vi "Get Integer Coefficients of Fixed-Point FIR Filter.vi"() -> ()   [LabVIEW 2023]
doc: "Demonstrates how to use the DFD Convert FXP to Integer VI to get integer coefficients of a fixed-point finite impulse response (FIR) filter.\n\nCompete the following steps to use this VI.\n1) Configure the <B>Coefficient Quantizer</B>.\n2) Run the VI.\n3) Observe the Coefficients Report.\n4) Examine the block diagram to learn how to get integer coefficients of a fixed-point FIR filter."
uses:
  <vilib>/addons/Digital Filter Design/_Objects.llb/DFD Quantization Settings.ctl
  <vilib>/addons/Digital Filter Design/_Objects.llb/DFD Quantization Sources.ctl
  <vilib>/addons/Digital Filter Design/FXPModel.llb/DFD FXP Quantize Coef (Advanced).vi
  <vilib>/addons/Digital Filter Design/FXPModel.llb/DFD FXP Get Quantizer (One).vi
  <vilib>/addons/Digital Filter Design/FXPLib.llb/DFD FXP to I16 (vector).vi
  <vilib>/addons/Digital Filter Design/NI_DigFilterLicensed.lvlib
panel:
  out "Coefficients Report":string
  out "Floating-Point FIR Coefficients":dbl[](array[numeric])
  out "Fixed-Point FIR Coefficients":dbl[](array[numeric])
  out "I16 FIR Coefficients":i16[](array[numeric])
  in  "Coefficients Quantizer":T1={"source"=7, "wl"=16, "iwl"=1, "overflow mode"=enum."Saturation", "rounding mode"=enum."Nearest", "signed?"=TRUE} {"source" items=["Coefficients a/k"=0, "Coefficients b/v"=7, "Input"=1, "Output"=2, "Multiplicand"=3, "Product"=4, "Sum"=5, "Delay"=6]}
  # "Select Help>>Show Context Help and move the cursor over the VI icon for more information."
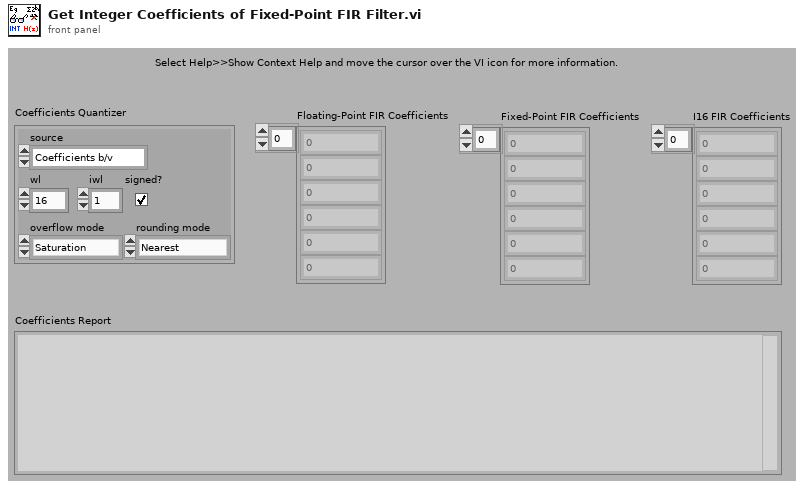
[diagram p1: front panel]
types:
  T1 = typedef "NI_DigFilterLicensed.lvlib/DFD Quantization Settings.ctl" = cluster{"source":T2, "wl":i16, "iwl":i16, "overflow mode":enum16{"Saturation", "Wrap"}, "rounding mode":enum16{"Nearest", "Truncation"}, "signed?":bool}
  T2 = typedef "NI_DigFilterLicensed.lvlib/DFD Quantization Sources.ctl" = u16
  T3 = typedef "NI_DigFilterLicensed.lvlib/DFD Filter Obj.ctl" = cluster{"mSRate_Fs":dbl, "mSRate_Version":string, "mSRate_Comments":string, "mSRate_OrgCoef":T4, "mSRate_CurCoef":T4, "mSRate_Quantized?":bool, "mSRate_QCoef":T4, "mSRate_QSettings":T6[], "mSRate_Order":i32, "mSRate_Scaling":cluster{"mSRate_ScaleByPowerOf2?":bool, "mSRate_ScaleType":T8}}
  T4 = typedef "NI_DigFilterLicensed.lvlib/DFD Filter Coef.ctl" = cluster{"type":T5, "gain":dbl, "coef a (k)":dbl[], "coef b (v)":dbl[]}
  T5 = typedef "NI_DigFilterLicensed.lvlib/DFD Filter Structure Type Selector.ctl" = enum16{"Undefined", "FIR Direct Form", "FIR Direct Form Transposed", "FIR Symmetric", "FIR Antisymmetric", "IIR Direct Form I", "IIR Direct Form I Transposed", "IIR Direct Form II", "IIR Direct Form II Transposed", "IIR Cascaded Second Order Sections Form I", "IIR Cascaded Second Order Sections Form I Transposed", "IIR Cascaded Second Order Sections Form II", "IIR Cascaded Second Order Sections Form II Transposed", "Lattice Allpass (basic sections)", "Lattice Allpass (one multiplier sections)", "Lattice Allpass (normalized sections)", "Lattice AR (basic sections)", "Lattice AR (one multiplier sections)", "Lattice AR (normalized sections)", "Lattice MA (minimum phase)", "Lattice MA (maximum phase)", "Lattice ARMA (basic sections)", "Lattice ARMA (one multiplier sections)", "Lattice ARMA (normalized sections)"}
  T6 = typedef "NI_DigFilterLicensed.lvlib/dfd_Internal Quantization Settings.ctl" = cluster{"source":T7, "wl":i16, "iwl":i16, "overflow mode":enum16{"Saturation", "Wrap"}, "rounding mode":enum16{"Nearest", "Truncation"}, "signed?":bool}
  T7 = typedef "NI_DigFilterLicensed.lvlib/dfd_Internal Quantization Srcs.ctl" = u16
  T8 = typedef "NI_DigFilterLicensed.lvlib/DFD Coef Norm Type.ctl" = enum16{"No Norm", "Time Domain 1-Norm", "Time Domain 2-Norm", "Time Domain Inf-Norm"}
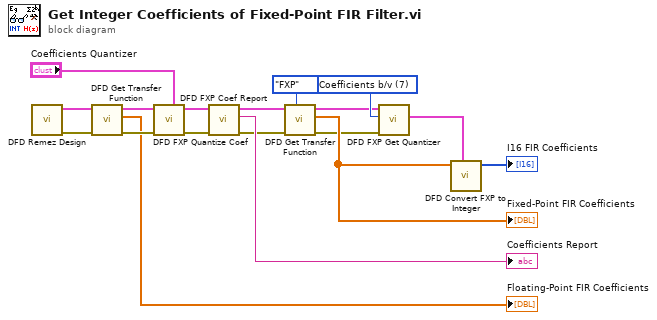
[diagram p0: block diagram]
diagram:
  w4 = T2 7 items=["Coefficients a/k"=0, "Coefficients b/v"=7, "Input"=1, "Output"=2, "Multiplicand"=3, "Product"=4, "Sum"=5, "Delay"=6] ("quantizer source")
  n1 = call <vilib>:"DFD Remez Design.vi"() -> ("error out"=w14:errorcluster, "filter out"=w15:T3)  [unwired: 7 in, 3 out]
  n2 = call <vilib>:"DFD Get Transfer Function.vi"("error in (no error)"=w14, "filter in"=w15) -> ("error out"=w12:errorcluster, "numerator"=→"Floating-Point FIR Coefficients":dbl[], "filter out"=w13:T3)  [unwired: 7 out]
  n3 = call-poly <vilib>:"DFD FXP Quantize Coef.vi"("coefficients b/v quantizer"="Coefficients Quantizer", "error in (no error)"=w12, "filter in"=w13) -> ("error out"=w9:errorcluster, "filter out"=w10:T3)  [unwired: 2 in, 5 out]
  n4 = call <vilib>:"DFD FXP Coef Report.vi"("error in (no error)"=w9, "filter in"=w10) -> ("error out"=w6:errorcluster, "coefficients report"=→"Coefficients Report":string, "filter out"=w7:T3)  [unwired: 7 out]
  n5 = call <vilib>:"DFD Get Transfer Function.vi"("type (FLP)"=enum16{"FLP", "FXP"}."FXP", "error in (no error)"=w6, "filter in"=w7) -> ("error out"=w5:errorcluster, "numerator"=w17:dbl[], "filter out"=w3:T3)  [unwired: 6 out]
  "Fixed-Point FIR Coefficients" <- w17
  n6 = call-poly <vilib>:"DFD FXP Get Quantizer.vi"("error in (no error)"=w5, "quantizer source"=w4, "filter in"=w3) -> ("quantizer"=w2:T1)  [unwired: 8 out]
  n7 = call-poly <vilib>:"DFD Convert FXP to Integer.vi"("quantization settings"=w2, "FXP values"=w17) -> ("I16 values"=→"I16 FIR Coefficients":i16[])  [unwired: 1 in, 8 out]
